vi "Configure Trigger D Slope.vi"(8 "error in (no error)":errorcluster, 9 "Slope (Rising Edge)":i32(ring) items=["Rising Edge", "Falling Edge"], 10 "Trigger (1)":i32=1, 11 "VISA resource name":refnum<visa-resource-name>) -> (0 "error out":errorcluster, 3 "VISA resource name out":refnum<visa-resource-name>)   [LabVIEW 2020, in "Rohde&Schwarz CMXP Base.lvlib"]
doc: "Specifies whether the rising edge or the falling edge of the trigger pulse is generated at the trigger event.\n\nThe setting applies to output trigger signals provided at the trigger connectors.\n\nAttributes:\nRSCMXPBASE_ATTR_SELECT_TRIGGER\nRSCMXPBASE_ATTR_TRIGGER_D_SLOPE\n\nRemote-control command:\nTRIGger:BASE:EXTD<n>:SLOPe"
uses:
  <instrlib>/Rohde&Schwarz CMXP Base/Rohde&Schwarz CMXP Base.lvlib
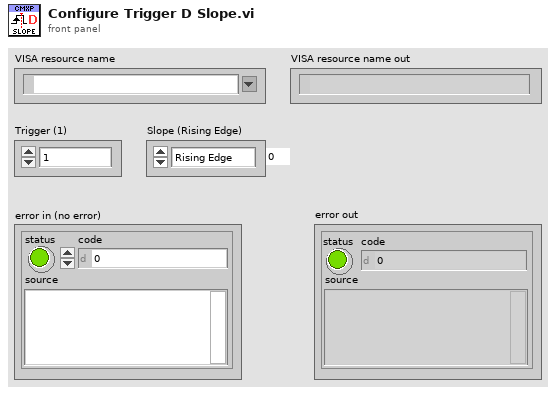
[diagram p1: front panel]
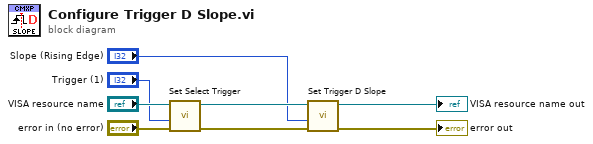
[diagram p0: block diagram]
diagram:
  n1 = call "Set Select Trigger"("error in (no error)"="error in (no error)", "Select Trigger (0)"="Trigger (1)", "instrument handle"="VISA resource name") -> ("error out"=w3:errorcluster, "instrument handle out"=w4:refnum<visa-resource-name>)  [unwired: 7 in]
  n2 = call "Set Trigger D Slope"("error in (no error)"=w3, "Trigger D Slope (0 - Rising Edge)"="Slope (Rising Edge)", "instrument handle"=w4) -> ("error out"=→"error out":errorcluster, "instrument handle out"=→"VISA resource name out":refnum<visa-resource-name>)  [unwired: 7 in]
